vi "根据列表的序号刷新列表名称.vi"(1 "总体列表名称数组输入":string[](array[string]), 2 "列表序号":u8[](array[numeric])) -> (0 "列表名称数组输出":string[](array[string]))   [LabVIEW 2015]
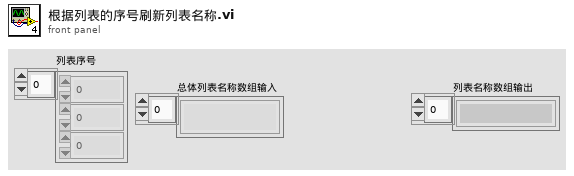
[diagram p1: front panel]
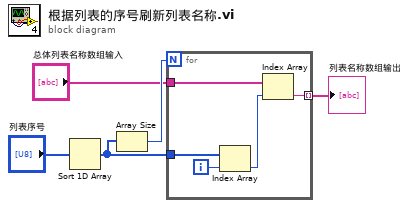
[diagram p0: block diagram]
diagram:
  n1 = Sort 1D Array(array="列表序号") -> (sorted array=w2:u8[])
  n2 = Array Size(array=w2) -> (size(s)=w4:i32)
  n3 = for {
    N: w4 -> [_]
    tunnel: "总体列表名称数组输入" -> [w10]
    tunnel: w2 -> [w6]
    tunnel: [w7] -> w5 mode=indexing
    i -> [w9]
    n4 = Index Array(array=w6, index=w9) -> (element=w8:u8)
    n5 = Index Array(array=w10, index=w8) -> (element=w7:string)
  }
  "列表名称数组输出" <- w5
